vi "jrg_binary_write.vi"(0 "Byte Stream File in":refnum<file>, 1 "nPts":i32, 2 "EODText":string, 3 "WaveformData":i16[](array[numeric]), 4 "prepend array or string size? (T)":bool, 5 "error in (no error)":errorcluster, 6 "AD Range":sgl, 7 "NBytes":i8, 8 "UserData":sgl, 9 "NBits":i8, 10 "Sample Rate":i32, 11 "byte order (0:big-endian, network order)":T1(ring), 12 "Polarity":i8, 13 "Version":i8) -> (14 "Byte Stream File out":refnum<file>, 19 "error out":errorcluster)   [LabVIEW 2014]
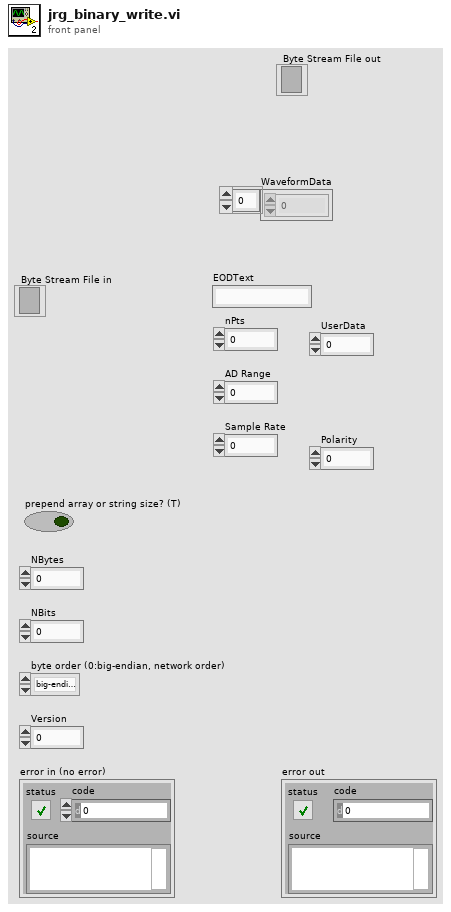
[diagram p1: front panel]
types:
  T1 = enum16{"big-endian, network order", "native, host order", "little-endian"}
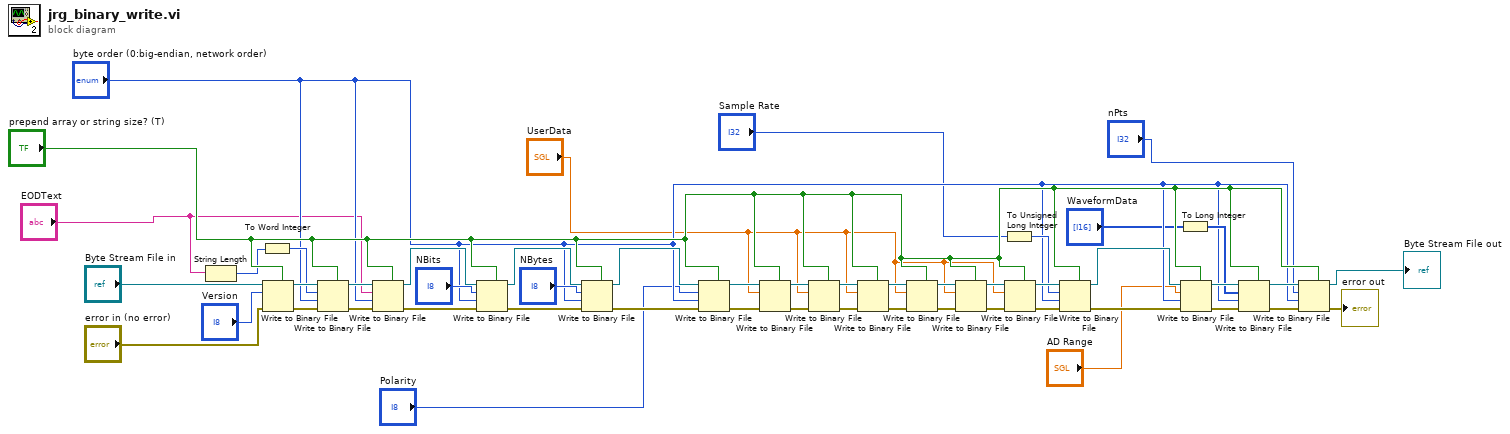
[diagram p0: block diagram]
diagram:
  n1 = String Length(string="EODText") -> (length=w8:i32)
  n2 = To Word Integer(number=w8) -> (16bit integer=w11:i16)
  n3 = Write to Binary File(file (use dialog)="Byte Stream File in", data="Version", error in="error in (no error)", 5:"prepend array or string size? (T)") -> (refnum out=w31:refnum<file>, error out=w30:errorcluster)  [unwired: 2 in, 1 out]
  n4 = Write to Binary File(file (use dialog)=w31, data=w11, error in=w30, 5:"prepend array or string size? (T)", 9:"byte order (0:big-endian, network order)") -> (refnum out=w18:refnum<file>, error out=w19:errorcluster)  [unwired: 1 in, 1 out]
  n5 = Write to Binary File(file (use dialog)=w18, data="EODText", error in=w19, 5:"prepend array or string size? (T)", 9:"byte order (0:big-endian, network order)") -> (refnum out=w32:refnum<file>, error out=w33:errorcluster)  [unwired: 1 in, 1 out]
  n6 = Write to Binary File(file (use dialog)=w32, data="NBits", error in=w33, 5:"prepend array or string size? (T)", 9:"byte order (0:big-endian, network order)") -> (refnum out=w28:refnum<file>, error out=w20:errorcluster)  [unwired: 1 in, 1 out]
  n7 = Write to Binary File(file (use dialog)=w28, data="NBytes", error in=w20, 5:"prepend array or string size? (T)", 9:"byte order (0:big-endian, network order)") -> (refnum out=w29:refnum<file>, error out=w21:errorcluster)  [unwired: 1 in, 1 out]
  n8 = Write to Binary File(file (use dialog)=w29, data="Polarity", error in=w21, 5:"prepend array or string size? (T)", 9:"byte order (0:big-endian, network order)") -> (refnum out=w47:refnum<file>, error out=w48:errorcluster)  [unwired: 1 in, 1 out]
  n9 = Write to Binary File(file (use dialog)=w47, data="UserData", error in=w48, 5:"prepend array or string size? (T)") -> (refnum out=w41:refnum<file>, error out=w36:errorcluster)  [unwired: 2 in, 1 out]
  n10 = Write to Binary File(file (use dialog)=w41, data="UserData", error in=w36, 5:"prepend array or string size? (T)") -> (refnum out=w42:refnum<file>, error out=w37:errorcluster)  [unwired: 2 in, 1 out]
  n11 = Write to Binary File(file (use dialog)=w42, data="UserData", error in=w37, 5:"prepend array or string size? (T)") -> (refnum out=w43:refnum<file>, error out=w38:errorcluster)  [unwired: 2 in, 1 out]
  n12 = Write to Binary File(file (use dialog)=w43, data="UserData", error in=w38, 5:"prepend array or string size? (T)") -> (refnum out=w44:refnum<file>, error out=w39:errorcluster)  [unwired: 2 in, 1 out]
  n13 = Write to Binary File(file (use dialog)=w44, data="UserData", error in=w39, 5:"prepend array or string size? (T)") -> (refnum out=w45:refnum<file>, error out=w40:errorcluster)  [unwired: 2 in, 1 out]
  n14 = To Unsigned Long Integer(number="Sample Rate") -> (unsigned 32bit integer=w14:u32)
  n15 = Write to Binary File(file (use dialog)=w45, data="UserData", error in=w40, 5:"prepend array or string size? (T)") -> (refnum out=w49:refnum<file>, error out=w50:errorcluster)  [unwired: 2 in, 1 out]
  n16 = Write to Binary File(file (use dialog)=w49, data=w14, error in=w50, 5:"prepend array or string size? (T)", 9:"byte order (0:big-endian, network order)") -> (refnum out=w22:refnum<file>, error out=w23:errorcluster)  [unwired: 1 in, 1 out]
  n17 = To Long Integer(number="WaveformData") -> (32bit integer=w15:i32[])
  n18 = Write to Binary File(file (use dialog)=w22, data="AD Range", error in=w23, 5:"prepend array or string size? (T)", 9:"byte order (0:big-endian, network order)") -> (refnum out=w24:refnum<file>, error out=w25:errorcluster)  [unwired: 1 in, 1 out]
  n19 = Write to Binary File(file (use dialog)=w24, data=w15, error in=w25, 5:"prepend array or string size? (T)", 9:"byte order (0:big-endian, network order)") -> (refnum out=w26:refnum<file>, error out=w27:errorcluster)  [unwired: 1 in, 1 out]
  n20 = Write to Binary File(file (use dialog)=w26, data="nPts", error in=w27, 5:"prepend array or string size? (T)", 9:"byte order (0:big-endian, network order)") -> (refnum out=→"Byte Stream File out":refnum<file>, error out=→"error out":errorcluster)  [unwired: 1 in, 1 out]
